vi "Main.vi"(11 "Module Admin":refnum<class "Delacor_lib_QMH_Module Admin.lvclass">) -> ()   [LabVIEW 2025, in "Acquisition.lvlib"]
doc: "This template is based off of the Queued Message Handler design pattern and the Queued Message Handler project template that ships with LabVIEW.\n\nThe main difference is that the queue is private to this module and communication between modules is performed via Broadcast and Request events.\n\nRequest events are wrapped in public API methods and are handled in the Event Handling Loop (EHL) of this VI. Any module can register for Broadcast events sent by this module. The EHL generates messages based on user interface actions.\n\nThe Message Handling Loop (MHL) processes messages generated by the EHL, or by other messages. The messages are string values, so new messages can be added easily to the Message Cases case structure in the MHL. Each message cluster can also provide an optional value for Message Data, which is a variant that can be converted to whatever message-specific data is required.\n_____\nBased on DQMH Project Template 4.0.0.47.\n_____\nBased on DQMH Dev Tools: Project Template 7.1.0.1503."
uses:
  Acquisition.lvlib
  <vilib>/Delacor/Delacor QMH/Libraries/Module Admin_class/Delacor_lib_QMH_Module Admin.lvclass
  Module Data--cluster.ctl
  Stop Argument--cluster.ctl
  <vilib>/Delacor/Delacor QMH/Libraries/Message Queue_class/Delacor_lib_QMH_Message Queue.lvclass/Delacor_lib_QMH_Message Queue.ctl
  <vilib>/Delacor/Delacor QMH/Libraries/Module Admin_class/Delacor_lib_QMH_Module Admin.lvclass/Delacor_lib_QMH_Module Admin.ctl
  Settings Editor/Update Application Settings (Reply Payload)--cluster.ctl
  Settings Editor/Settings--cluster.ctl
  Settings Editor/Test Meta Data.ctl
  Start Acquiring (Reply Payload)--cluster.ctl
  <vilib>/Utility/miscctls.llb/LVPointTypeDef.ctl
  Start Acquiring Argument--cluster.ctl
  <vilib>/DAQmx/read.llb/DAQmx Read (Analog 1D Wfm NChan NSamp).vi
  <vilib>/Analysis/baseanly.llb/Mean (DBL).vi
  <vilib>/Delacor/Delacor QMH/Libraries/Message Queue_class/Delacor_lib_QMH_Enqueue Message (Single).vi
  <vilib>/Delacor/Delacor QMH/Libraries/Module Admin_class/Delacor_lib_QMH_Get External Launch.vi
  <vilib>/DAQmx/miscellaneous.llb/DAQmx Fill In Error Info.vi
  <vilib>/Delacor/Delacor QMH/Libraries/Message Queue_class/Delacor_lib_QMH_Message Queue.lvclass
  Settings Editor/Settings Editor.lvlib
  Logger/Logger.lvlib
  <vilib>/Analysis/NI_AALBase.lvlib
  <vilib>/ptbypt/NI_PtbyPt.lvlib
panel:
  out "Settings":T1
  out "error out":errorcluster
  # "This is a headless module. Show its panel to confirm that the Settings are updated correctly and other debugging tasks. Use the Settings Editor to change the settings for this module."
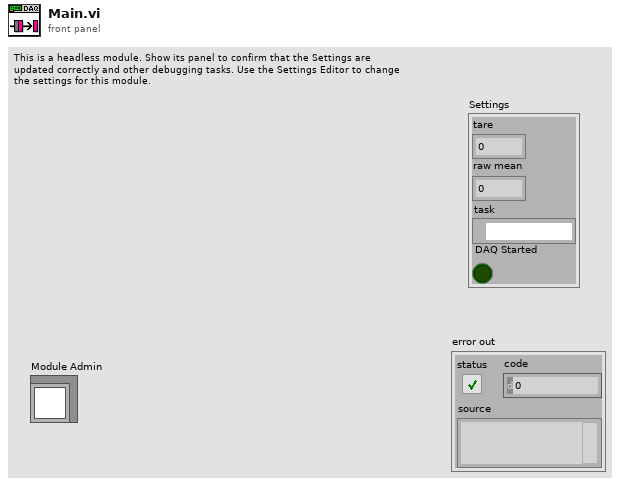
[diagram p1: front panel]
types:
  T1 = typedef "Acquisition.lvlib/Module Data--cluster.ctl" = cluster{"tare":dbl, "raw mean":dbl, "task":refnum<k21>, "DAQ Started":bool}
  T2 = typedef "Settings Editor.lvlib/Broadcast Events--cluster.ctl" = cluster{"Module Did Init":refnum<user-event>, "Status Updated":refnum<user-event>, "Error Reported":refnum<user-event>, "Module Did Stop":refnum<user-event>, "Update Module Execution Status":refnum<user-event>, "Application Settings Updated":refnum<user-event>}
  T3 = typedef "Acquisition.lvlib/Request Events--cluster.ctl" = cluster{"Stop Module":refnum<user-event>, "Show Panel":refnum<user-event>, "Hide Panel":refnum<user-event>, "Get Module Execution Status":refnum<user-event>, "Show Diagram":refnum<user-event>, "Stop Acquiring":refnum<user-event>, "Wakeup Helper Loop":refnum<user-event>, "Change Settings":refnum<user-event>, "Tare":refnum<user-event>, "Start Acquiring":refnum<user-event>}
  T4 = typedef "Acquisition.lvlib/Start Acquiring (Reply Payload)--cluster.ctl" = cluster{"error":errorcluster}
  T5 = enum32{"invalid lock state", "Not Locked", "Locked (No Password)", "Password-protected"}
  T6 = typedef "Acquisition.lvlib/Stop Argument--cluster.ctl" = cluster{"Origin":string, "Exit via Stop Module Req?":bool, "Wait for Module to stop?":bool}
  T7 = typedef "Settings Editor.lvlib/Update Application Settings (Reply Payload)--cluster.ctl" = cluster{"Settings":T8, "error":errorcluster}
  T8 = typedef "Settings Editor.lvlib/Settings--cluster.ctl" = cluster{"Log File Base Path":path, "Meta Data":T9, "DAQ Settings":cluster{"physical channel":string, "minimum value":dbl, "maximum value":dbl, "number of samples":i32, "rate":dbl, "custom scale name":string}}
  T9 = typedef "Settings Editor.lvlib/Test Meta Data.ctl" = cluster{"Operator":string, "Job Number":string, "Part Number":string}
  T10 = typedef "LVPointTypeDef.ctl" = cluster{"Horizontal":i16, "Vertical":i16}
  T11 = enum32{"Invalid", "Standard", "Closed", "Hidden", "Minimized", "Maximized"}
  T12 = typedef "Acquisition.lvlib/Start Acquiring Argument--cluster.ctl" = cluster{"Wait Notifier":refnum<notifier>, "wait for reply":bool}
  T13 = cluster{"physical channel":string, "minimum value":dbl, "maximum value":dbl, "number of samples":i32, "rate":dbl, "custom scale name":string}
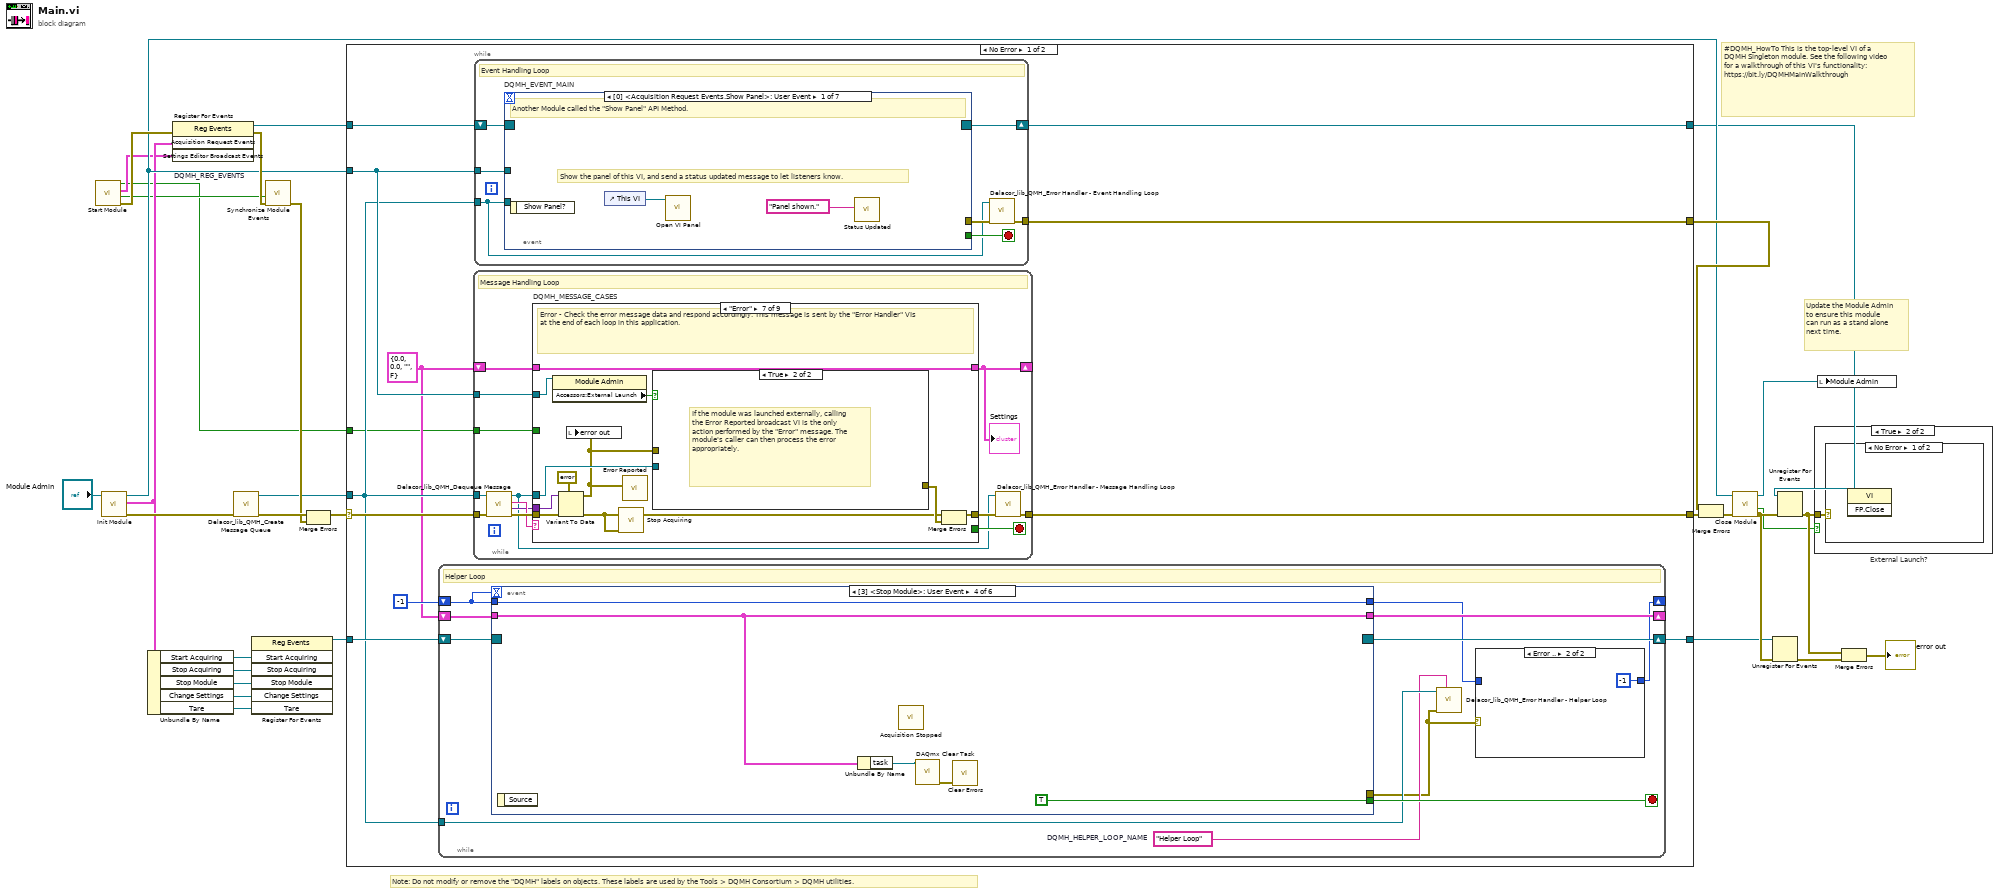
[diagram p0: block diagram]
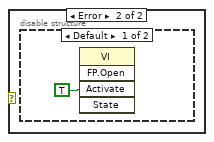
[diagram p3: hidden frame]
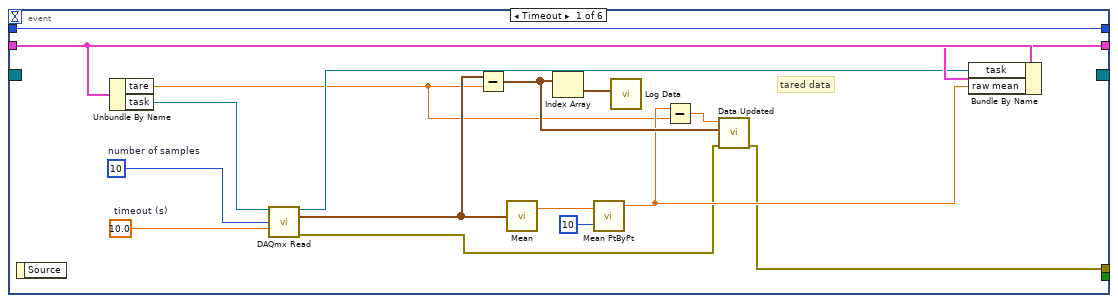
[diagram p6: hidden frame]
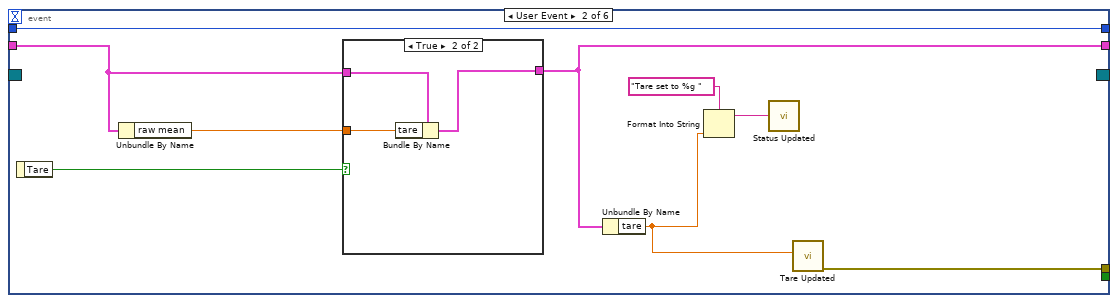
[diagram p7: hidden frame]
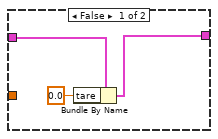
[diagram p8: hidden frame]
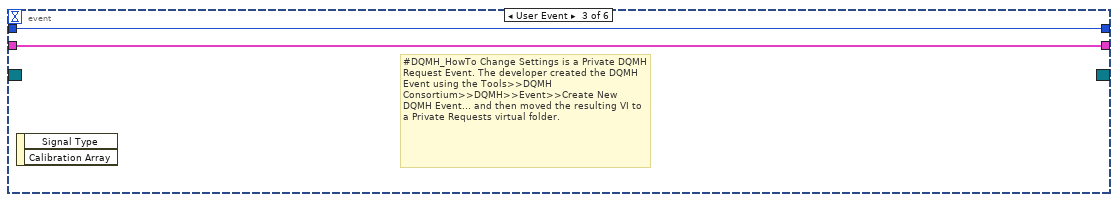
[diagram p9: hidden frame]
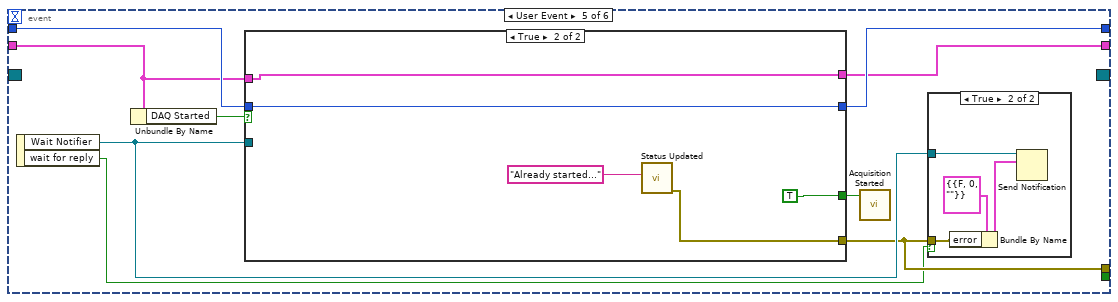
[diagram p10: hidden frame]
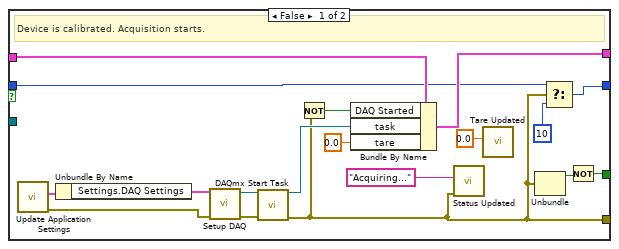
[diagram p12: hidden frame]
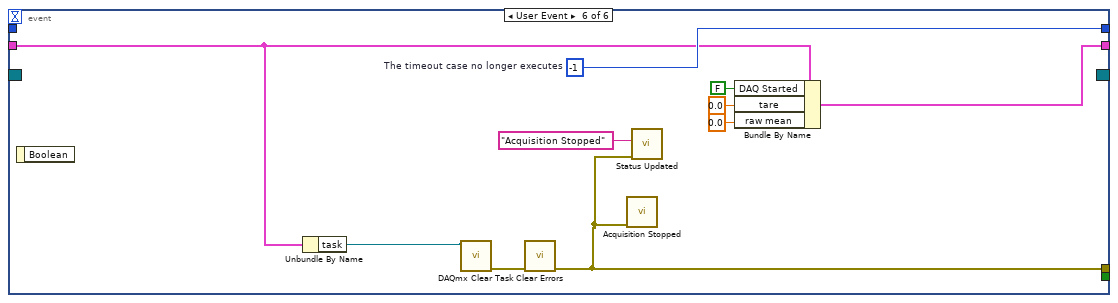
[diagram p13: hidden frame]
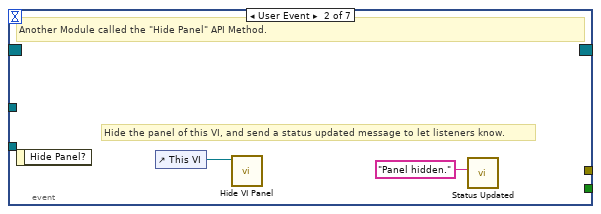
[diagram p14: hidden frame]
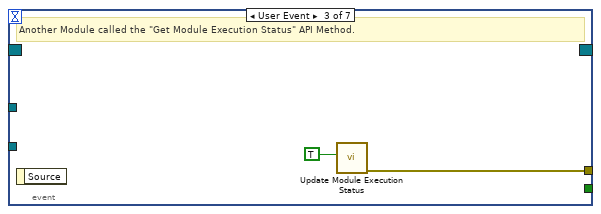
[diagram p15: hidden frame]
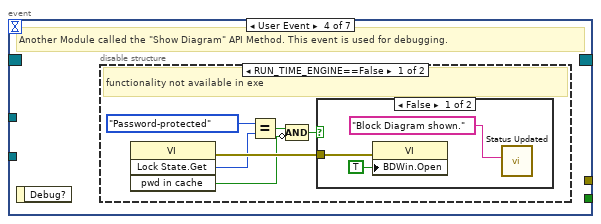
[diagram p16: hidden frame]
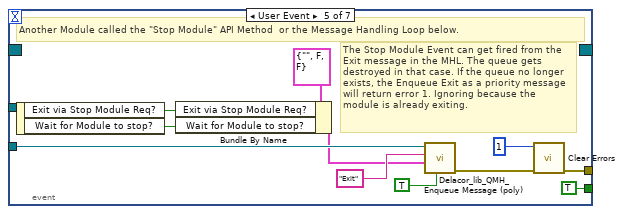
[diagram p19: hidden frame]
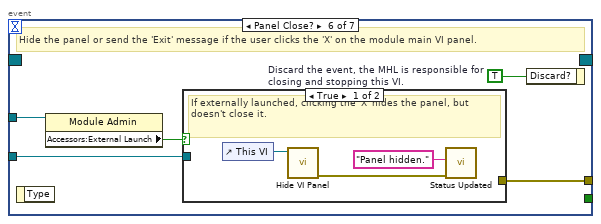
[diagram p20: hidden frame]
diagram:
  # "#DQMH_HowTo This is the top-level VI of a DQMH Singleton module. See the following video for a walkthrough of this VI's functionality: https://bit.ly/DQMHMainWalkthrough"
  # "Note: Do not modify or remove the \"DQMH\" labels on objects. These labels are used by the Tools > DQMH Consortium > DQMH utilities."
  # "Update the Module Admin to ensure this module can run as a stand alone next time."
  n1 = call "Start Module.vi"() -> ("error out"=w24:errorcluster, "Wait for Event Sync?"=w5:bool, "Settings Editor Broadcast Events"=w6:T2, "Module Was Already Running?"=w1:bool)  [unwired: 7 in, 1 out]
  n2 = call "Init Module.vi"("Singleton Module Admin in"="Module Admin") -> ("error out"=w30:errorcluster, "Acquisition Request Events"=w11:T3, "Singleton Module Admin out"=w18:refnum<class "Delacor_lib_QMH_Module Admin.lvclass">)  [unwired: 8 in]
  n3 = Unbundle By Name(w11) -> ("Start Acquiring"=w7:refnum<user-event>, "Stop Acquiring"=w10:refnum<user-event>, "Stop Module"=w9:refnum<user-event>, "Change Settings"=w4:refnum<user-event>, "Tare"=w3:refnum<user-event>)
  n4 = register-events "DQMH_REG_EVENTS"(error in=w24, w11, w6) -> (reference out=w16:refnum<event-registration>, error out=w23:errorcluster)  [unwired: 1 in]
  n5 = call <vilib>:"Delacor_lib_QMH_Create Message Queue.vi"("error in"=w30) -> ("error out"=w26:errorcluster, "Message Queue"=w15:refnum<class "Delacor_lib_QMH_Message Queue.lvclass">)  [unwired: 9 in]
  n6 = register-events(w7, w10, w9, w4, w3) -> (reference out=w8:refnum<event-registration>)  [unwired: 2 in, 1 out]
  n7 = call "Synchronize Module Events.vi"("error in"=w23, "Wait for Event Sync?"=w5) -> ("error out"=w22:errorcluster)  [unwired: 9 in]
  n8 = Merge Errors(w26, w22) -> (w25:errorcluster)
  n9 = case shown="No Error" w25 {
    selector: w25 -> [w41 w303]
    tunnel: [w43 w302] -> w31
    tunnel: [w40 w301] -> w17
    tunnel: w16 -> [w39 w301]
    tunnel: w15 -> [w35 w294]
    tunnel: [w42 _] -> w29
    tunnel: w18 -> [w38 w297]
    tunnel: w8 -> [w36 w296]
    tunnel: [w33 w296] -> w2
    tunnel: w1 -> [w32 w295]
    frame No Error {
      w34 = T1 {"tare"=0.0, "raw mean"=0.0, "task"="", "DAQ Started"=FALSE} ("Data Cluster")
      n10 = while {
        shift-right: [w44] -> _
        shift-left: -1 -> [w54]
        tunnel: w35 -> [w48]
        shift-right: [w51] -> _
        shift-left: w34 -> [w50]
        shift-right: [w49] -> w33
        shift-left: w36 -> [w53]
        stop <- w52 stop-if-true
        w47 = "Helper Loop"  # DQMH_HELPER_LOOP_NAME
        # "Helper Loop"
        n11 = event shown="[3] <Stop Module>: User Event" {
          selector: w53 -> [_ _ _ _ _ _]
          dyn-events: [_ _ _ _ _ _] -> w49
          timeout: w54 -> [_ _ _ _ _ _]
          tunnel: [w73 w81 w90 w95 w104 w141] -> w45
          tunnel: w54 -> [w73 w81 w90 w95 w99 _]
          tunnel: [_ _ _ TRUE _ _] -> w52
          tunnel: [w58 w82 _ _ w102 w132] -> w46
          tunnel: [w68 w80 w89 w92 w97 w137] -> w51
          tunnel: w50 -> [w69 w79 w89 w92 w98 w138]
          event Timeout {
            w71 = 10  # number of samples
            w72 = 10.0  # timeout (s)
            # "tared data"
            n12 = event-data() -> ()  [unwired: 1 in, 1 out]
            n13 = Unbundle By Name(w69) -> ("tare"=w59:dbl, "task"=w70:refnum<k21>)
            n14 = call-poly <vilib>:"DAQmx Read.vi"("task/channels in"=w70, "number of samples per channel"=w71, "timeout"=w72) -> ("task out"=w67:refnum<k21>, "data"=w62:waveform(dbl)[], "error out"=w57:errorcluster)  [unwired: 10 in]
            n15 = Subtract(x=w62, y=w59) -> (x-y=w63:waveform(dbl)[])
            n16 = call-poly <vilib>:"Mean.vi"("X"=w62) -> ("mean"=w65:dbl)  [unwired: 1 out]
            n17 = Index Array(array=w63) -> (element=w66:waveform(dbl))  [unwired: 1 in]
            n18 = call <vilib>:"Mean PtByPt.vi"("x"=w65, "sample length"=10) -> ("mean"=w61:dbl)  [unwired: 2 in, 1 out]
            n19 = call "Log Data.vi"("Waveform"=w66) -> ()  [unwired: 10 in, 1 out]
            n20 = Subtract(x=w61, y=w59) -> (x-y=w60:dbl)
            n21 = call "Data Updated.vi"("error in"=w57, "Graph Data"=w63, "Numeric"=w60) -> ("error out"=w58:errorcluster)  [unwired: 8 in]
            n22 = Bundle By Name(cluster=w69, "task"=w67, "raw mean"=w61) -> (w68:T1)
          }
          event User Event {
            n23 = event-data() -> ("Tare"=w75:bool)  [unwired: 1 in]
            n24 = Unbundle By Name(w79) -> ("raw mean"=w76:dbl)
            n25 = case shown="True" w75 {
              tunnel: [w84 w87] -> w80
              tunnel: w79 -> [w85 w88]
              tunnel: w76 -> [_ w86]
              frame False {
                n26 = Bundle By Name(cluster=w85, "tare"=0.0) -> (w84:T1)
              }
              frame True {
                n27 = Bundle By Name(cluster=w88, "tare"=w86) -> (w87:T1)
              }
            }
            n28 = Unbundle By Name(w80) -> ("tare"=w74:dbl)
            n29 = Format Into String(format string="Tare set to %g " ("Status"), w74) -> (resulting string=w77:string)  [unwired: 2 in, 1 out]
            n30 = call "Status Updated.vi"("Status"=w77) -> ()  [unwired: 10 in, 1 out]
            n31 = call "Tare Updated.vi"("Tare Offset"=w74) -> ("error out"=w82:errorcluster)  [unwired: 10 in]
          }
          event User Event {
            # "#DQMH_HowTo Change Settings is a Private DQMH Request Event. The developer created the DQMH Event using the Tools>>DQMH Consortium>>DQMH>>Event>>Create New DQMH Event... and then moved the resulting VI to a Private Requests virtual folder."
            n32 = event-data() -> ()  [unwired: 1 in, 2 out]
          }
          event User Event {
            n33 = event-data() -> ()  [unwired: 1 in, 1 out]
            n34 = Unbundle By Name(w92) -> ("task"=w93:refnum<k21>)
            n35 = call "Acquisition Stopped.vi"() -> ()  [unwired: 11 in, 1 out]
            n36 = call <vilib>:"DAQmx Clear Task.vi"("task in"=w93) -> ("error out"=w91:errorcluster)  [unwired: 14 in]
            n37 = call <vilib>:"Clear Errors.vi"("error in (no error)"=w91) -> ()  [unwired: 5 in, 2 out]
          }
          event User Event {
            n38 = event-data() -> ("Wait Notifier"=w103:refnum<notifier>, "wait for reply"=w101:bool)  [unwired: 1 in]
            n39 = Unbundle By Name(w98) -> ("DAQ Started"=w100:bool)
            n40 = case shown="True" w100 {
              tunnel: [w112 w130] -> w104
              tunnel: w103 -> [_ _]
              tunnel: [w111 w129] -> w102
              tunnel: w99 -> [w114 w130]
              tunnel: w98 -> [w124 w128]
              tunnel: [w122 w128] -> w97
              tunnel: [w109 TRUE ("Success")] -> w96
              frame False {
                # "Device is calibrated. Acquisition starts."
                n41 = call "Update Application Settings.vi"() -> ("error out"=w115:errorcluster, "Reply Payload"=w117:T7)  [unwired: 9 in, 1 out]
                n42 = Unbundle By Name(w117) -> ("Settings.DAQ Settings"=w116:T13)
                n43 = call "Setup DAQ.vi"("error in"=w115, "Cluster"=w116) -> ("error out"=w121:errorcluster, "task out"=w126:refnum<k21>)  [unwired: 8 in]
                n44 = call <vilib>:"DAQmx Start Task.vi"("task/channels in"=w126, "error in"=w121) -> ("task out"=w120:refnum<k21>, "error out"=w111:errorcluster)  [unwired: 12 in]
                n45 = Not(x=w111) -> (.not. x?=w123:bool)
                n46 = Bundle By Name(cluster=w124, "DAQ Started"=w123, "task"=w120, "tare"=0.0) -> (w122:T1)
                n47 = call "Status Updated.vi"("error in"=w111, "Status"="Acquiring...") -> ()  [unwired: 9 in, 1 out]
                n48 = call "Tare Updated.vi"("Tare Offset"=0.0) -> ()  [unwired: 10 in, 1 out]
                n49 = Unbundle(w111) -> ("status"=w110:bool)  [unwired: 2 out]
                n50 = Select(t=w114, s=w111, f=10) -> (s? t:f=w112:i32)
                n51 = Not(x=w110) -> (.not. x?=w109:bool)
              }
              frame True {
                n52 = call "Status Updated.vi"("Status"="Already started...") -> ("error out"=w129:errorcluster)  [unwired: 10 in]
              }
            }
            n53 = call "Acquisition Started.vi"("Success"=w96) -> ()  [unwired: 10 in, 1 out]
            n54 = case shown="True" w101 {
              tunnel: w103 -> [_ w106]
              tunnel: w102 -> [_ w105]
              frame False {
              }
              frame True {
                n55 = Bundle By Name(cluster=T4 {"error"={"status"=FALSE, "code"=0, "source"=""}} ("Start Acquisition (Reply Payload)"), "error"=w105) -> (w108:T4)
                n56 = Send Notification(notification=w108, notifier=w106) -> ()  [unwired: 1 in, 2 out]
              }
            }
          }
          event User Event {
            w141 = -1  # The timeout case no longer executes
            n57 = event-data() -> ()  [unwired: 1 in, 1 out]
            n58 = Unbundle By Name(w138) -> ("task"=w140:refnum<k21>)
            n59 = call <vilib>:"DAQmx Clear Task.vi"("task in"=w140) -> ("error out"=w135:errorcluster)  [unwired: 14 in]
            n60 = call <vilib>:"Clear Errors.vi"("error in (no error)"=w135) -> ("error out"=w132:errorcluster)  [unwired: 5 in, 1 out]
            n61 = call "Acquisition Stopped.vi"("error in"=w132) -> ()  [unwired: 10 in, 1 out]
            n62 = call "Status Updated.vi"("error in"=w132, "Status"="Acquisition Stopped") -> ()  [unwired: 9 in, 1 out]
            n63 = Bundle By Name(cluster=w138, "DAQ Started"=FALSE, "tare"=0.0, "raw mean"=0.0) -> (w137:T1)
          }
        }
        n64 = call-dynamic "Delacor_lib_QMH_Error Handler - Helper Loop.vi"("Error Debug"=w47, "error in"=w46, "Message Queue in"=w48) -> ()  [unwired: 7 in, 2 out]
        n65 = case shown="Error .." w46 {
          tunnel: w45 -> [w55 _]
          tunnel: [w55 -1 ("The timeout case no longer executes")] -> w44
          frame No Error {
          }
          frame Error {
          }
        }
      }
      n66 = while {
        tunnel: w35 -> [w196]
        shift-right: [w200] -> _
        shift-left: w34 -> [w201]
        tunnel: w41 -> [w204]
        tunnel: [w202] -> w43
        tunnel: w38 -> [w194]
        tunnel: w32 -> [w193]
        stop <- w199 stop-if-true
        # "Message Handling Loop"
        n67 = call-dynamic "Delacor_lib_QMH_Dequeue Message.vi"("error in"=w204, "Message Queue in"=w196) -> ("error out"=w203:errorcluster, "Message Data"=w197:variant, "Message"=w198:string, "Message Queue out"=w195:refnum<class "Delacor_lib_QMH_Message Queue.lvclass">)  [unwired: 6 in]
        n68 = case "DQMH_MESSAGE_CASES" shown="\"Error\"" w198 {
          selector: w198 -> [_ _ _ _ _ _ _ _ w289]
          tunnel: w195 -> [_ _ _ _ _ _ w253 w275 _]
          tunnel: w203 -> [w224 w228 w237 w243 w246 w248 w259 w281 w292]
          tunnel: [w210 w228 w229 w238 w245 w248 w256 w276 w293] -> w205
          tunnel: w201 -> [w206 w227 w230 w241 w244 w247 w255 w267 w290]
          tunnel: [w206 w227 w230 w241 w244 w247 w255 w267 w290] -> w200
          tunnel: [_ _ _ _ _ _ _ w274 _] -> w199
          tunnel: w197 -> [_ _ w236 w242 _ _ w254 w273 _]
          tunnel: w194 -> [w216 _ _ _ _ _ w252 w268 _]
          tunnel: w193 -> [_ _ _ _ _ _ _ w266 _]
          frame "Initialize" {
            # "Initialize - Any operation that needs to be done before the module can receive messages. Synchronize Caller Events.vi will inform Start Module.vi that the module has launched and is ready to receive messages. Module Did Init.vi will broadcast that the module initialized."
            n69 = call "Synchronize Caller Events.vi"("error in"=w224, "Singleton Module Admin in"=w216) -> ("error out"=w208:errorcluster, "Singleton Module Admin out"=w213:refnum<class "Delacor_lib_QMH_Module Admin.lvclass">)  [unwired: 8 in]
            n70 = call "Update Application Settings.vi"("wait for reply (T)"=TRUE) -> ("error out"=w207:errorcluster)  [unwired: 8 in, 2 out]
            n71 = property on="Property Node" class="Module Admin"(reference=w213) -> ("Accessors:External Launch"=w220:bool)  [unwired: 1 in, 2 out]
            n72 = Select(t=T11."Hidden" ("State"), s=w220, f=T11."Standard" ("State")) -> (s? t:f=w217:T11)
            n73 = Merge Errors(w208, w207) -> (w209:errorcluster)
            n74 = call "Module Name--constant.vi"() -> ("Module Name"=w223:string)  [unwired: 11 in]
            n75 = property on="Property Node" class="VI"("Front Panel.Title"=w223) -> (reference out=w222:refnum<vi>, error out=w226:errorcluster)  [unwired: 2 in]
            n76 = invoke on="Invoke Node" class="VI" method="FP.Open"(reference=w222, error in=w226, "State"=w217) -> (reference out=w221:refnum<vi>, error out=w225:errorcluster)  [unwired: 2 in, 3 out]
            n77 = call "Module Name--constant.vi"() -> ("Module Name"=w214:string)  [unwired: 11 in]
            n78 = invoke on="Invoke Node" class="VI" method="FP.Center"(reference=w221, error in=w225) -> ()  [unwired: 1 in, 3 out]
            n79 = property on="Pane" class="Pane"("Origin"=T10 {"Horizontal"=0, "Vertical"=0}) -> ()  [unwired: 2 in, 2 out]
            n80 = call "Module Did Init.vi"("error in"=w209, "Initialized?"=TRUE, "Origin"=w214) -> ("error out"=w210:errorcluster)  [unwired: 8 in]
          }
          frame "---Module Specific---" {
            # "Separator -- The following cases handle messages specific to this Module."
          }
          frame "Start Acquiring" {
            # "Requests Acquisition Module to start acquiring."
            n81 = Variant To Data(error in=w237, type=T12 {"Wait Notifier"=refnum, "wait for reply"=FALSE} ("Start Acquisition Argument"), Variant=w236) -> (data=w234:T12, error out=w229:errorcluster)
            n82 = Unbundle By Name(w234) -> ("Wait Notifier"=w233:refnum<notifier>)
            n83 = Bundle By Name(cluster=T4 {"error"={"status"=FALSE, "code"=0, "source"=""}} ("Start Acquisition (Reply Payload)"), "error"=w229) -> (w232:T4)
            n84 = Send Notification(notification=w232, notifier=w233) -> ()  [unwired: 1 in, 2 out]
          }
          frame "Update Settings" {
            # "Send the Change Settings event to the helper loop."
            # "The Settings Editor broadcasted that the settings have changed."
            n85 = Variant To Data(error in=w243, type=T7 {"Settings"={"Log File Base Path"=path "", "Meta Data"={"Operator"="", "Job Number"="", "Part Number"=""}, "DAQ Settings"={"physical channel"="cDAQ9181-1913300Mod1/ai0", "minimum value"=0.0, "maximum value"=94400.0, "number of samples"=10, "rate"=125.0, "custom scale name"="Pressure"}}, "error"={"status"=FALSE, "code"=0, "source"=""}} ("Settings Updated Argument"), Variant=w242) -> (error out=w238:errorcluster)  [unwired: 1 out]
            n86 = call "Status Updated.vi"("error in"=w238, "Status"="Settings Updated") -> ()  [unwired: 9 in, 1 out]
          }
          frame "---Copy This Frame---" {
            # "Duplicate this frame when creating new messages.  Change this comment in the duplicated frame to describe this message."
            n87 = Merge Errors(w246) -> (w245:errorcluster)
          }
          frame "---Exit and Error Handling---" {
            # "Separator - The following cases handle errors and exit messages."
          }
          frame "Error" {
            # "Error - Check the error message data and respond accordingly. This message is sent by the \"Error Handler\" VIs at the end of each loop in this application."
            n88 = property on="Property Node" class="Module Admin"(reference=w252) -> ("Accessors:External Launch"=w251:bool)  [unwired: 1 in, 2 out]
            n89 = Variant To Data(error in=w259, type=errorcluster {"status"=FALSE, "code"=0, "source"=""} ("error constant"), Variant=w254) -> (data=w250:errorcluster, error out=w249:errorcluster)
            n90 = local write "error out"(w250) -> ()
            n91 = call "Stop Acquiring.vi"("error in"=w249) -> ()  [unwired: 10 in, 1 out]
            n92 = call "Error Reported.vi"("Error"=w250) -> ()  [unwired: 10 in, 1 out]
            n93 = case shown="True" w251 {
              tunnel: [w264 _] -> w257
              tunnel: w253 -> [w262 _]
              tunnel: w250 -> [w263 _]
              frame False {
                n94 = disable-structure shown="DQMH_Disable_SEH==TRUE" {
                  disable-tunnel: w263 -> [w265 _]
                  frame condition #0 (active) {
                    # "If the module is running standalone, then pop up an error dialog and call the \"Exit\" message."
                    n95 = call <vilib>:"Simple Error Handler.vi"("error in (no error)"=w265) -> ()  [unwired: 4 in, 5 out]
                  }
                  frame condition #1 {
                    # "To prevent the Simple Error Handler VI from being loaded (e.g. when deploying to a Real-Time target), add the Conditional Disable Symbol \"DQMH_Disable_SEH\" to your project and set it to TRUE."
                  }
                }
                n96 = call-poly <vilib>:"Delacor_lib_QMH_Enqueue Message (poly).vi"("Priority Message? (F)"=TRUE, "Message"="Exit", "Message Queue in"=w262) -> ("error out"=w264:errorcluster)  [unwired: 7 in, 1 out]
              }
              frame True {
                # "If the module was launched externally, calling the Error Reported broadcast VI is the only action performed by the \"Error\" message. The module's caller can then process the error appropriately."
              }
            }
            n97 = Merge Errors(w249, w257) -> (w256:errorcluster)
          }
          frame "Exit" {
            w274 = TRUE  # Stop the VI
            # "Release the message queue reference"
            # "Exit - Exit the application."
            n98 = Variant To Data(error in=w281, type=T6 {"Origin"="", "Exit via Stop Module Req?"=FALSE, "Wait for Module to stop?"=FALSE} ("Stop Argument"), Variant=w273) -> (data=w270:T6, error out=w278:errorcluster)
            n99 = call <vilib>:"Clear Errors.vi"("error in (no error)"=w278, "specific error code to clear (0: all)"=91 ("91: not all Exit messages will have an argument")) -> ("error out"=w280:errorcluster)  [unwired: 4 in, 1 out]
            n100 = control-ref of="This VI"() -> (w269:refnum<vi>)
            n101 = call "Handle Exit.vi"("Stop Argument"=w270, "Admin in"=w268, "VI reference"=w269) -> ("error out"=w277:errorcluster)  [unwired: 7 in, 1 out]
            n102 = call-dynamic "Delacor_lib_QMH_Release Message Queue.vi"("error in"=w280, "Message Queue"=w275) -> ("error out"=w279:errorcluster)  [unwired: 9 in]
            n103 = case "Settings Editor was\nalready running?" shown="False" w266 {
              frame False {
                n104 = call "Module Name--constant.vi"() -> ("Module Name"=w283:string)  [unwired: 11 in]
                n105 = call "Stop Module.vi"("Wait for Module to Stop? (F)"=TRUE, "Origin"=w283) -> ()  [unwired: 9 in, 1 out]
              }
              frame True {
                # "Another Module stops the Settings Editor"
              }
            }
            n106 = Merge Errors(w279, w277) -> (w276:errorcluster)
            n107 = call "Error Reported.vi"("Error"=w276) -> ()  [unwired: 10 in, 1 out]
          }
          frame Default {
            # "'Default' case only runs if there is a message that isn't defined in any of the other cases.  Output a programming error."
            n108 = call "Module Name--constant.vi"() -> ("Module Name"=w288:string)  [unwired: 11 in]
            n109 = Format Into String(format string="The invalid message string \"%s\" was received in the Message Handling Loop for module \"%s\".", w289, w288) -> (resulting string=w286:string)  [unwired: 2 in, 1 out]
            n110 = call <vilib>:"Error Cluster From Error Code.vi"("show call chain? (False)"=TRUE, "error message (\"\")"=w286, "error code (0)"=1) -> ("error out"=w291:errorcluster)  [unwired: 6 in]
            n111 = Merge Errors(w292, w291) -> (w293:errorcluster)
          }
        }
        "Settings" <- w200
        n112 = call-dynamic "Delacor_lib_QMH_Error Handler - Message Handling Loop.vi"("error in"=w205, "Message Queue in"=w195) -> ("dup error in"=w202:errorcluster)  [unwired: 8 in, 1 out]
      }
      n113 = while {
        tunnel: w35 -> [w142]
        shift-right: [w145] -> w40
        shift-left: w39 -> [w146]
        tunnel: [w147] -> w42
        tunnel: w38 -> [w143]
        stop <- w144 stop-if-true
        # "Event Handling Loop"
        n114 = event "DQMH_EVENT_MAIN" shown="[0] <Acquisition Request Events.Show Panel>: User Event" {
          selector: w146 -> [_ _ _ _ _ _ _]
          dyn-events: [_ _ _ _ _ _ _] -> w145
          timeout: _ -> [_ _ _ _ _ _ _]
          tunnel: [_ _ _ _ TRUE ("Discard?") _ _] -> w144
          tunnel: w142 -> [_ _ _ _ w170 w177 w190]
          tunnel: [_ _ w154 _ w173 w179 w192] -> w148
          tunnel: w143 -> [_ _ _ _ _ w176 _]
          event User Event {
            # "Show the panel of this VI, and send a status updated message to let listeners know."
            # "Another Module called the \"Show Panel\" API Method."
            n115 = event-data() -> ()  [unwired: 1 in, 1 out]
            n116 = control-ref of="This VI"() -> (w150:refnum<vi>)
            n117 = call "Open VI Panel.vi"("VI"=w150) -> ()  [unwired: 10 in, 1 out]
            n118 = call "Status Updated.vi"("Status"="Panel shown." ("format string")) -> ()  [unwired: 10 in, 1 out]
          }
          event User Event {
            # "Hide the panel of this VI, and send a status updated message to let listeners know."
            # "Another Module called the \"Hide Panel\" API Method."
            n119 = event-data() -> ()  [unwired: 1 in, 1 out]
            n120 = control-ref of="This VI"() -> (w152:refnum<vi>)
            n121 = call "Hide VI Panel.vi"("VI"=w152) -> ()  [unwired: 10 in, 1 out]
            n122 = call "Status Updated.vi"("Status"="Panel hidden." ("format string")) -> ()  [unwired: 10 in, 1 out]
          }
          event User Event {
            # "Another Module called the \"Get Module Execution Status\" API Method."
            n123 = event-data() -> ()  [unwired: 1 in, 1 out]
            n124 = call "Update Module Execution Status.vi"("Running?"=TRUE) -> ("error out"=w154:errorcluster)  [unwired: 10 in]
          }
          event User Event {
            # "Another Module called the \"Show Diagram\" API Method. This event is used for debugging."
            n125 = event-data() -> ()  [unwired: 1 in, 1 out]
            n126 = disable-structure shown="RUN_TIME_ENGINE==False" {
              frame condition #0 (active) {
                # "functionality not available in exe"
                n127 = invoke on="Invoke Node" class="VI" method="Lock State.Get"() -> (error out=w160:errorcluster, "Get Lock State"=w159:T5, "pwd in cache"=w156:bool)  [unwired: 4 in, 1 out]
                n128 = Equal?(x=T5."Password-protected", y=w159) -> (x = y?=w157:bool)
                n129 = Compound Arithmetic op=AND(w157, invert w156) -> (w155:bool)
                n130 = case shown="False" w155 {
                  tunnel: w160 -> [w163 _]
                  frame False {
                    n131 = property on="Property Node" class="VI"(error in=w163, "BDWin.Open"=TRUE ("Block Diagram Window:Open")) -> ()  [unwired: 1 in, 2 out]
                    n132 = call "Status Updated.vi"("Status"="Block Diagram shown." ("format string")) -> ()  [unwired: 10 in, 1 out]
                  }
                  frame True {
                    # "Password-protected VI, and the password is not in the cache. Do not show the diagram."
                  }
                }
              }
              frame condition #1 {
              }
            }
          }
          event User Event {
            # "The Stop Module Event can get fired from the Exit message in the MHL. The queue gets destroyed in that case. If the queue no longer exists, the Enqueue Exit as a priority message will return error 1. Ignoring because the module is already exiting."
            # "Another Module called the \"Stop Module\" API Method  or the Message Handling Loop below."
            n133 = event-data() -> ("Exit via Stop Module Req?"=w166:bool, "Wait for Module to stop?"=w165:bool)  [unwired: 1 in]
            n134 = Bundle By Name(cluster=T6 {"Origin"="", "Exit via Stop Module Req?"=FALSE, "Wait for Module to stop?"=FALSE} ("Stop Argument"), "Exit via Stop Module Req?"=w166, "Wait for Module to stop?"=w165) -> (w164:T6)
            n135 = call-poly <vilib>:"Delacor_lib_QMH_Enqueue Message (poly).vi"("Priority Message? (F)"=TRUE, "Message Data"=w164, "Message"="Exit", "Message Queue in"=w170) -> ("error out"=w174:errorcluster)  [unwired: 6 in, 1 out]
            n136 = call <vilib>:"Clear Errors.vi"("error in (no error)"=w174, "specific error code to clear (0: all)"=1) -> ("error out"=w173:errorcluster)  [unwired: 4 in, 1 out]
          }
          event Panel Close? {
            w178 = TRUE  # Discard the event, the MHL is responsible for closing and stopping this VI.
            # "Hide the panel or send the 'Exit' message if the user clicks the 'X' on the module main VI panel."
            n137 = event-data() -> ()  [unwired: 1 in, 1 out]
            n138 = property on="Property Node" class="Module Admin"(reference=w176) -> ("Accessors:External Launch"=w175:bool)  [unwired: 1 in, 2 out]
            n139 = case shown="True" w175 {
              tunnel: w177 -> [_ w185]
              tunnel: [_ w186] -> w179
              frame True {
                # "If externally launched, clicking the 'X' hides the panel, but doesn't close it."
                n140 = control-ref of="This VI"() -> (w182:refnum<vi>)
                n141 = call "Hide VI Panel.vi"("VI"=w182) -> ("error out"=w180:errorcluster)  [unwired: 10 in]
                n142 = call "Status Updated.vi"("error in"=w180, "Status"="Panel hidden." ("format string")) -> ()  [unwired: 9 in, 1 out]
              }
              frame False {
                # "If run as a stand-alone VI, clicking the panel 'X' stops the VI."
                n143 = call-poly <vilib>:"Delacor_lib_QMH_Enqueue Message (poly).vi"("Priority Message? (F)"=TRUE, "Message"="Exit", "Message Queue in"=w185) -> ("error out"=w186:errorcluster)  [unwired: 7 in, 1 out]
              }
            }
            n144 = event-data ("Event Filter Node")("Discard?"=w178) -> ()  [unwired: 1 in, 1 out]
          }
          event User Event {
            n145 = event-data() -> ("Settings"=w187:T8)  [unwired: 1 in]
            n146 = Bundle By Name(cluster=T7 {"Settings"={"Log File Base Path"=path "", "Meta Data"={"Operator"="", "Job Number"="", "Part Number"=""}, "DAQ Settings"={"physical channel"="cDAQ9181-1913300Mod1/ai0", "minimum value"=0.0, "maximum value"=94400.0, "number of samples"=10, "rate"=125.0, "custom scale name"="Pressure"}}, "error"={"status"=FALSE, "code"=0, "source"=""}} ("Settings Updated Argument"), "Settings"=w187) -> (w189:T7)
            n147 = call-poly <vilib>:"Delacor_lib_QMH_Enqueue Message (poly).vi"("Message Data"=w189, "Message"="Update Settings", "Message Queue in"=w190) -> ("error out"=w192:errorcluster)  [unwired: 7 in, 1 out]
          }
        }
        n148 = call-dynamic "Delacor_lib_QMH_Error Handler - Event Handling Loop.vi"("error in"=w148, "Message Queue in"=w142) -> ("dup error in"=w147:errorcluster)  [unwired: 8 in, 1 out]
      }
    }
    frame Error {
      # "Synchronize Caller Events.vi will inform Start Module.vi that the module has launched and will let the code calling Start Module.vi register for broadcasts and would permit the caller receive the broadcast that an error occurred at launch time."
      n149 = call "Synchronize Caller Events.vi"("Singleton Module Admin in"=w297) -> ("error out"=w304:errorcluster)  [unwired: 9 in, 1 out]
      n150 = call-dynamic "Delacor_lib_QMH_Release Message Queue.vi"("error in"=w303, "Message Queue"=w294) -> ("error out"=w302:errorcluster)  [unwired: 9 in]
      n151 = call "Module Name--constant.vi"() -> ("Module Name"=w300:string)  [unwired: 11 in]
      n152 = case "Settings Editor was\nalready running?" shown="False" w295 {
        frame False {
          n153 = call "Module Name--constant.vi"() -> ("Module Name"=w307:string)  [unwired: 11 in]
          n154 = call "Stop Module.vi"("Wait for Module to Stop? (F)"=TRUE, "Origin"=w307) -> ()  [unwired: 9 in, 1 out]
        }
        frame True {
          # "Another Module is\nin charge of stopping Settings Editor"
        }
      }
      n155 = Format Into String(format string="An error occurred during initialization. %s is no longer running.", w300) -> (resulting string=w298:string)  [unwired: 2 in, 1 out]
      n156 = Merge Errors(w302, w304) -> (w305:errorcluster)
      n157 = call "Error Reported.vi"("Additional Information"=w298, "Error"=w305) -> ()  [unwired: 9 in, 1 out]
    }
  }
  n158 = Merge Errors(w29, w31) -> (w28:errorcluster)
  n159 = call "Close Module.vi"("error in"=w28, "Module Admin in"=w18) -> ("error out"=w21:errorcluster, "External Launch"=w12:bool, "Module Admin out"=w13:refnum<class "Delacor_lib_QMH_Module Admin.lvclass">)  [unwired: 7 in]
  n160 = Unregister For Events(event registration refnum=w2, error in=w21) -> (error out=w19:errorcluster)
  n161 = Unregister For Events(event registration refnum=w17, error in=w21) -> (error out=w27:errorcluster)
  n162 = case "External Launch?" shown="True" w12 {
    tunnel: w27 -> [_ w308]
    frame False {
    }
    frame True {
      n163 = case shown="No Error" w308 {
        frame No Error {
          n164 = invoke on="Invoke Node" class="VI" method="FP.Close"() -> ()  [unwired: 3 in, 3 out]
        }
        frame Error {
          n165 = disable-structure shown="Default" {
            frame condition #0 (active) {
              n166 = invoke class="VI" method="FP.Open"("Activate"=TRUE ("Activate?")) -> ()  [unwired: 4 in, 5 out]
            }
            frame condition #1 {
              # "Don't show panel on error if running inside a built EXE."
            }
          }
        }
      }
    }
  }
  n167 = local write "Module Admin"(w13) -> ()
  n168 = Merge Errors(w27, w19) -> (→"error out":errorcluster)
